vi "SoS_Kr_2024.vi"(4 "Frequency (Hz)":dbl=20000.0, 5 "CO2 content (ppm)":dbl=542.0, 6 "xw molar fraction water vapor":dbl=0.01309 format="%.6g", 7 "Pressure (Pa)":dbl=99951.0 format="%.1f", 8 "Temperature (K)":dbl=293.4405 format="%.4g", 9 "Type of air":i32(listbox)=4) -> (0 "Kr":dbl, 1 "Heat capacity & virial corr speed of sound [m/s]":dbl format="%.4f", 3 "Heat capacity, virial and relax corr speed of sound [m/s]":dbl format="%.4g")   [LabVIEW 2016]
panel:
  out "Rel strength N2":dbl=0.00012703722717918718 format="%#_6e"
  out "Rel strength O2":dbl=0.0006753922167312215 format="%#_6e"
  out "Kr (ppm)":dbl format="%.1f"
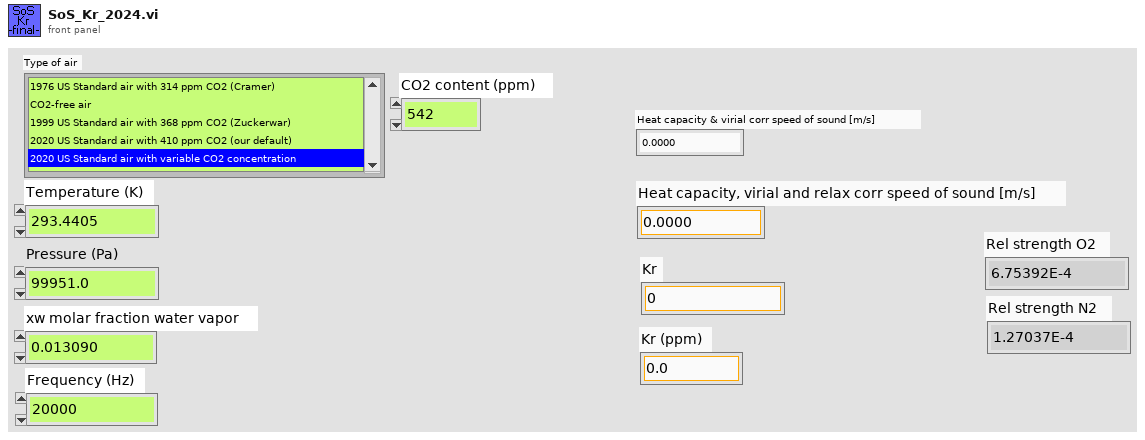
[diagram p1: front panel]
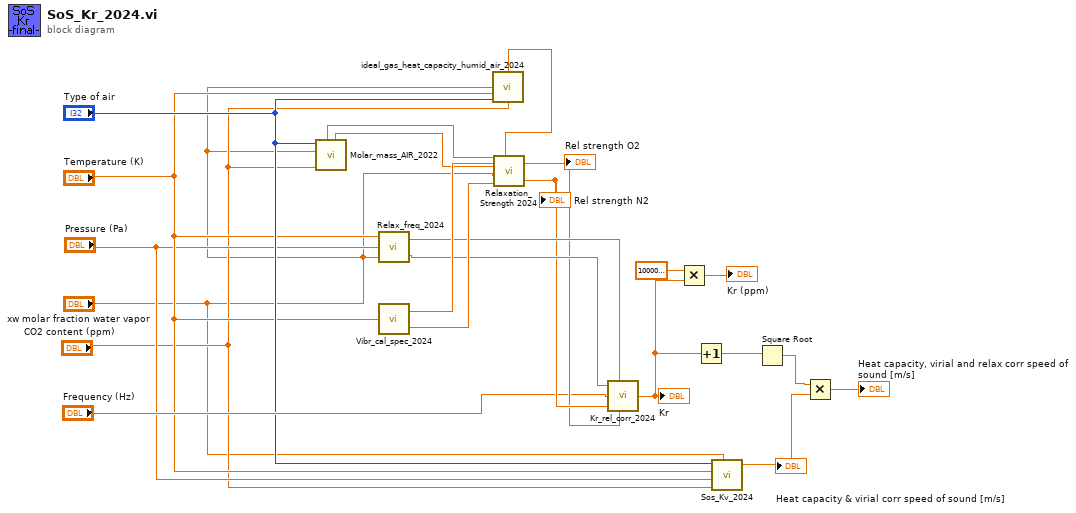
[diagram p0: block diagram]
diagram:
  n1 = call "Molar_mass_AIR_2022.vi"("CO2 content (ppm)"="CO2 content (ppm)", "xw molar fraction of water vapor"="xw molar fraction water vapor", "Type of air"="Type of air") -> ("xN2"=w17:dbl, "xO2"=w18:dbl)  [unwired: 7 out]
  n2 = call "Relax_freq_2024.vi"("H2O molar fraction"="xw molar fraction water vapor", "Pressure [Pa]"="Pressure (Pa)", "Temperature [K]"="Temperature (K)") -> ("Relax freq N2"=w14:dbl, "Relax freq O2"=w15:dbl)
  n3 = call "Vibr_cal_spec_2024.vi"("Temperature [K]"="Temperature (K)") -> ("Cvib O2 [J mol-1 K-1]"=w22:dbl, "Cvib N2 [J mol-1 K-1]"=w21:dbl)
  n4 = call "ideal_gas_heat_capacity_humid_air_2024.vi"("molar fraction of water vapor"="xw molar fraction water vapor", "Temperature [K]"="Temperature (K)", "Type of air"="Type of air", "CO2 content (ppm)"="CO2 content (ppm)") -> ("Cp0/R humid air"=w16:dbl)  [unwired: 2 in, 9 out]
  n5 = call "Relaxation_Strength 2024.vi"("Cp0 humid air / R"=w16, "C vib O2"=w22, "C vib N2"=w21, "xw molar fraction water vapor"="xw molar fraction water vapor", "N2 molar fraction Dry"=w17, "O2 molar fraction Dry"=w18) -> ("Rel strength N2"=w13:dbl, "Rel strength O2"=w12:dbl)
  "Rel strength O2" <- w12
  "Rel strength N2" <- w13
  n6 = call "Kr_rel_corr_2024.vi"("N2 rel freq / Hz"=w14, "O2 rel freq / Hz"=w15, "Frequency / Hz"="Frequency (Hz)", "N2 rel strength"=w13, "O2 rel strength"=w12) -> ("Kr"=w9:dbl)
  "Kr" <- w9
  n7 = Multiply(x=1000000.0, y=w9) -> (x*y=→"Kr (ppm)":dbl)
  n8 = Increment(x=w9) -> (x+1=w10:dbl)
  n9 = call "Sos_Kv_2024.vi"("Type of air"="Type of air", "Temperature (K)"="Temperature (K)", "Pressure (Pa)"="Pressure (Pa)", "CO2 content (ppm)"="CO2 content (ppm)", "xw molar fraction water vapor"="xw molar fraction water vapor") -> ("Sos Kv (m/s)"=w6:dbl)  [unwired: 1 in, 1 out]
  "Heat capacity & virial corr speed of sound [m/s]" <- w6
  n10 = Square Root(x=w10) -> (sqrt(x)=w20:dbl)
  n11 = Multiply(x=w20, y=w6) -> (x*y=→"Heat capacity, virial and relax corr speed of sound [m/s]":dbl)
